vi "make plots for obrit angle panel.vi"(10 "time axis in hrs":bool, 11 "orbit fit":T1[](array[typedef])) -> (0 "ellipse fit":T2 {"deg/hr pred" format="%0.2f"}, 1 "deg/hr vs time":cluster{dbl[], dbl[]}, 2 "minor/major axes vs time":cluster{dbl[], dbl[]}[](array[cluster]), 3 "graphs (t, theta, theta_fit, dtheta_dt)":cluster{dbl[], dbl[]}[](array[cluster]), 4 "orbit is":enum16{"clockwise", "counterclockwise"}(ring), 5 "angle":dbl, 7 "deg/hr":dbl format="%0.2f")   [LabVIEW 2017]
uses:
  typedefs/orbit parameters with crossing info.ctl
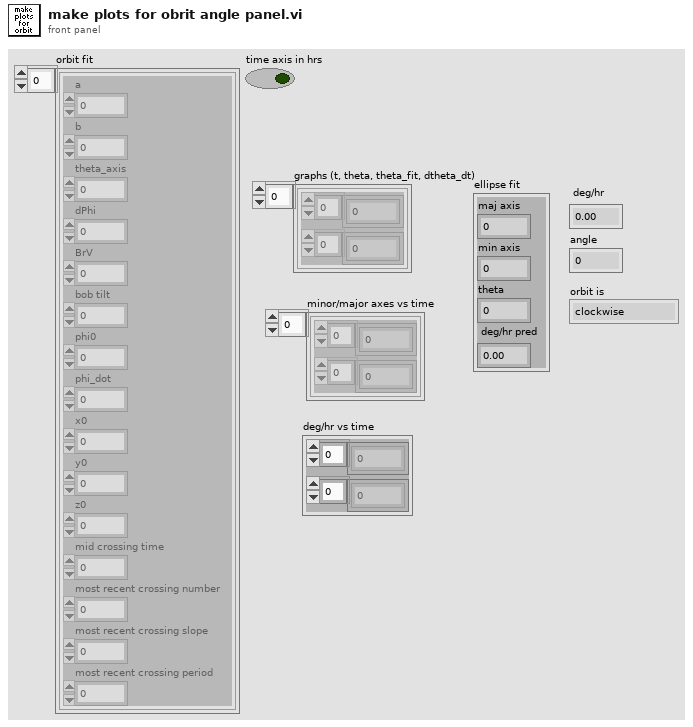
[diagram p1: front panel]
types:
  T1 = typedef "orbit parameters with crossing info.ctl" = cluster{"a":dbl, "b":dbl, "theta_axis":dbl, "dPhi":dbl, "BrV":dbl, "bob tilt":dbl, "phi0":dbl, "phi_dot":dbl, "x0":dbl, "y0":dbl, "z0":dbl, "mid crossing time":dbl, "most recent crossing number":dbl, "most recent crossing slope":dbl, "most recent crossing period":dbl}
  T2 = cluster{"maj axis":dbl, "min axis":dbl, "theta":dbl, "deg/hr pred":dbl}
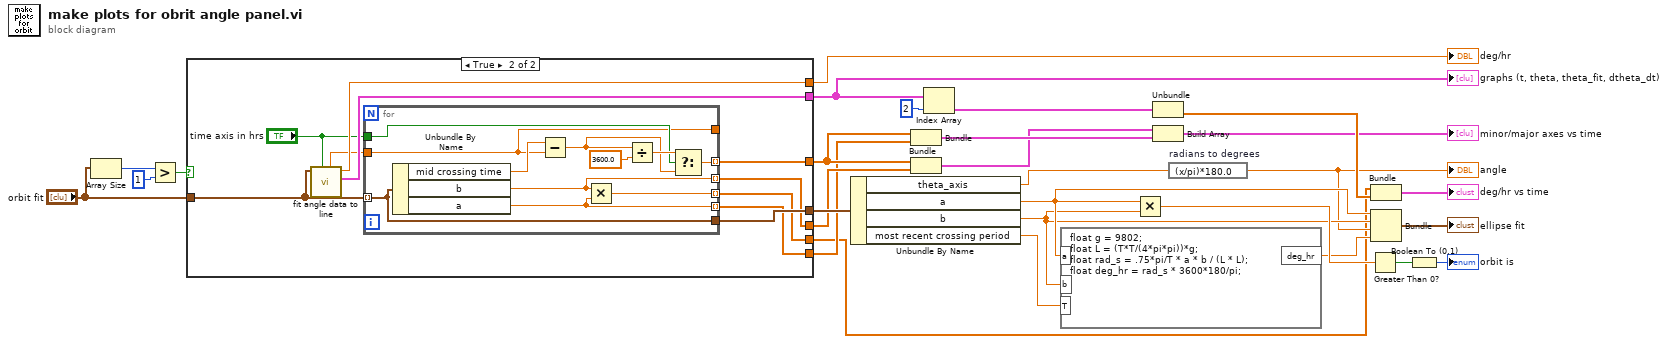
[diagram p0: block diagram]
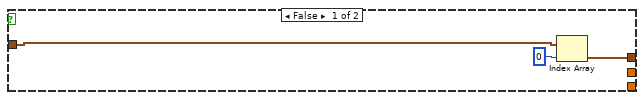
[diagram p2: hidden frame]
diagram:
  n1 = Array Size(array="orbit fit") -> (size(s)=w11:i32)
  n2 = Greater?(x=w11, y=1) -> (0:w9:bool)
  n3 = case shown="True" w9 {
    tunnel: "orbit fit" -> [w31 w39]
    tunnel: [_ w41] -> w7
    tunnel: [_ w40] -> w6
    tunnel: [w29 w37] -> w5
    tunnel: [_ w35] -> w4
    tunnel: [_ w34] -> w3
    tunnel: [_ w33] -> w2
    tunnel: [_ w32] -> w1
    frame False {
      n4 = Index Array(array=w31, index=0) -> (element=w29:T1)
    }
    frame True {
      n5 = call "fit angle data to line.vi"("hrs"="time axis in hrs", "orbit fit"=w39) -> ("graphs (t, theta, theta_fit, dtheta_dt)"=w41:cluster{dbl[], dbl[]}[], "deg/hr"=w40:dbl, "tmin"=w38:dbl)  [unwired: 6 in, 1 out]
      n6 = for {
        tunnel: [w49] -> w35 mode=indexing
        tunnel: [w47] -> w34 mode=indexing
        tunnel: [w43] -> w37
        tunnel: [w46] -> w32 mode=indexing
        tunnel: "time axis in hrs" -> [w45]
        tunnel: [w44] -> w33 mode=indexing
        tunnel: [w42] -> _
        tunnel: w39 -> [w43] mode=indexing
        tunnel: w38 -> [w42]
        n7 = Unbundle By Name(w43) -> ("mid crossing time"=w52:dbl, "b"=w47:dbl, "a"=w44:dbl)
        n8 = Subtract(x=w52, y=w42) -> (x-y=w48:dbl)
        n9 = Multiply(x=w47, y=w44) -> (x*y=w46:dbl)
        n10 = Divide(x=w48, y=3600.0) -> (x/y=w50:dbl)
        n11 = Select(t=w50, s=w45, f=w48) -> (s? t:f=w49:dbl)
      }
    }
  }
  "deg/hr" <- w6
  "graphs (t, theta, theta_fit, dtheta_dt)" <- w7
  n12 = Unbundle By Name(w5) -> ("theta_axis"=w26:dbl, "a"=w24:dbl, "b"=w23:dbl, "most recent crossing period"=w22:dbl)
  n13 = Bundle(w4, w2) -> (w28:cluster{dbl[], dbl[]})  [unwired: 1 in]
  n14 = Bundle(w4, w3) -> (w20:cluster{dbl[], dbl[]})  [unwired: 1 in]
  n15 = Index Array(array=w7, index=2) -> (element=w19:cluster{dbl[], dbl[]})
  n16 = formula code="float g = 9802;\nfloat L = (T*T/(4*pi*pi))*g;\nfloat rad_s = .75*pi/T * a * b / (L * L);\nfloat deg_hr = rad_s * 3600*180/pi;"("a"=w24, "b"=w23, "T"=w22) -> ("deg_hr"=w21:dbl)
  n17 = Multiply(x=w24, y=w23) -> (x*y=w27:dbl)
  n18 = Unbundle(w19) -> (w25:dbl[])  [unwired: 1 out]
  n19 = Build Array(w20, w28) -> (→"minor/major axes vs time":cluster{dbl[], dbl[]}[])
  n20 = expression code="(x/pi)*180.0" "radians to degrees"(w26) -> (w12:dbl)
  "angle" <- w12
  n21 = Greater Than 0?(x=w27) -> (x > 0?=w14:bool)
  n22 = Bundle(w1, w25) -> (→"deg/hr vs time":cluster{dbl[], dbl[]})  [unwired: 1 in]
  n23 = Bundle("a"=w24, "b"=w23, "theta_axis"=w12, w21) -> (→"ellipse fit":cluster{"a":dbl, "b":dbl, "theta_axis":dbl, dbl})  [unwired: 1 in]
  n24 = Boolean To (0,1)(Boolean=w14) -> (0, 1=→"orbit is":i16)
